vi "TCPclient.vi"(6 "Input Command":string=" 1 1 1 1 0 1 1 0 0 0", 7 "Port #":i32=23) -> (0 "Telnet error":errorcluster, 2 "Command and Results":string, 3 "Open Connection":string, 5 "IP Address":string="192.168.1.158")   [LabVIEW 2018]
doc: "The Telnet Line Client VI uses the Telnet VIs to simulate a simple Telnet Window."
uses:
  Global 2.vi
panel:
  out "First":bool=TRUE
  # "Netburner TCP/IO Routine"
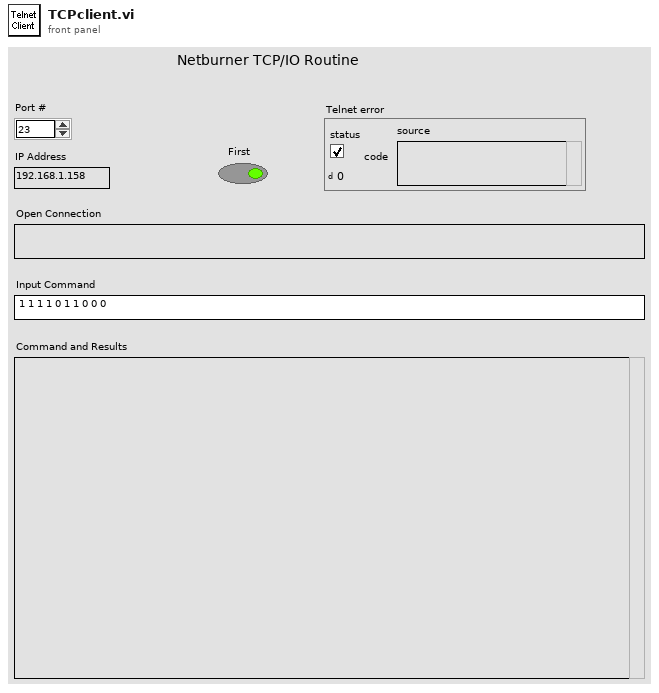
[diagram p1: front panel]
types:
  T1 = enum16{"Standard", "Buffered", "CRLF", "Immediate"}
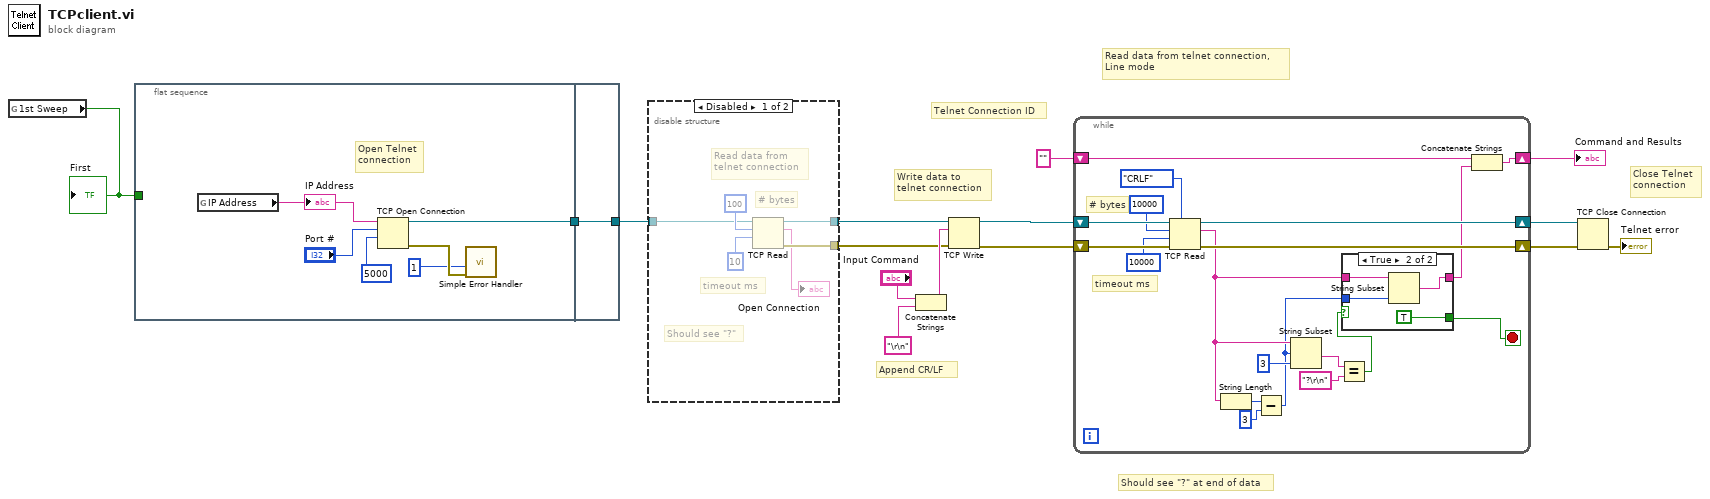
[diagram p0: block diagram]
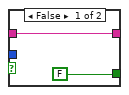
[diagram p2: hidden frame]
diagram:
  # "Should see \"?\" at end of data"
  # "Read data from telnet connection, \nLine mode"
  # "Append CR/LF"
  # "Telnet Connection ID"
  # "Write data to \ntelnet connection"
  # "Close Telnet \nconnection"
  n1 = global read "Global 2.vi" "1st Sweep"() -> (w10:bool)
  "First" <- w10
  n2 = flat-sequence {
    tunnel: w10 -> [_]
    tunnel: [w21] -> w9
    tunnel: w9 -> [w22]
    tunnel: [w22] -> w8
    frame #0 {
      # "Open Telnet\nconnection"
      n3 = global read "Global 2.vi" "IP Address"() -> (w19:string)
      "IP Address" <- w19
      n4 = TCP Open Connection(address=w19, remote port or service name="Port #", timeout ms (60000)=5000) -> (connection ID=w21:refnum<k5>, error out=w17:errorcluster)  [unwired: 2 in]
      n5 = call <vilib>:"Simple Error Handler.vi"("type of dialog (OK msg:1)"=1, "error in (no error)"=w17) -> ()  [unwired: 3 in, 5 out]
    }
    frame #1 {
    }
  }
  n6 = disable-structure shown="Disabled" {
    disable-tunnel: [w28 _] -> w12
    disable-tunnel: [w24 w29] -> w11
    disable-tunnel: w8 -> [w23 w29]
    frame Disabled {
      # "timeout ms"
      # "# bytes"
      # "Should see \"?\""
      # "Read data from \ntelnet connection"
      n7 = TCP Read(connection ID=w23, bytes to read=100, 9:10 ("timeout ms (25000)")) -> (connection ID out=w24:refnum<k5>, data out=→"Open Connection":string, error out=w28:errorcluster)  [unwired: 2 in]
    }
    frame Enabled {
    }
  }
  n8 = Concatenate Strings("Input Command", "\r\n") -> (w13:string)
  n9 = TCP Write(connection ID=w11, data in=w13, error in (no error)=w12) -> (connection ID out=w6:refnum<k5>, error out=w7:errorcluster)  [unwired: 1 in, 1 out]
  n10 = while {
    shift-right: [w43] -> w4
    shift-left: w7 -> [w48]
    shift-right: [w44] -> w5
    shift-left: w6 -> [w47]
    shift-right: [w32] -> w1
    shift-left: "" ("data out") -> [w33]
    stop <- w40 stop-if-true
    # "timeout ms"
    # "# bytes"
    n11 = TCP Read(connection ID=w47, bytes to read=10000, error in (no error)=w48, 7:T1."CRLF" ("mode (standard)"), 9:10000 ("timeout ms (25000)")) -> (connection ID out=w44:refnum<k5>, data out=w38:string, error out=w43:errorcluster)
    n12 = String Length(string=w38) -> (length=w37:i32)
    n13 = Subtract(x=w37, y=3) -> (x-y=w30:i32)
    n14 = String Subset(string=w38, offset (0)=w30, length (rest)=3 ("length (rest)")) -> (substring=w34:string)
    n15 = Equal?(x=w34, y="?\r\n") -> (x = y?=w41:bool)
    n16 = case shown="True" w41 {
      tunnel: [FALSE TRUE] -> w40
      tunnel: w38 -> [w49 w53]
      tunnel: [w49 w51] -> w31
      tunnel: w30 -> [_ w52]
      frame False {
      }
      frame True {
        n17 = String Subset(string=w53, length (rest)=w52) -> (substring=w51:string)  [unwired: 1 in]
      }
    }
    n18 = Concatenate Strings(w33, w31) -> (w32:string)
  }
  "Command and Results" <- w1
  n19 = TCP Close Connection(connection ID=w5, error in (no error)=w4) -> (error out=→"Telnet error":errorcluster)  [unwired: 1 in, 1 out]
